vi "Finding Sensor Center.vi"() -> ()   [LabVIEW 2021]
uses:
  Classes/Workspace/Workspace.ctl
  Classes/Workspace/Component/Component Tray.lvclass
  Classes/Controller/Controller.lvclass
  Classes/Workspace/Fixture.lvclass
panel:
  out "error out":errorcluster
  in  "error in (no error)":errorcluster
  out "Workspace":T1
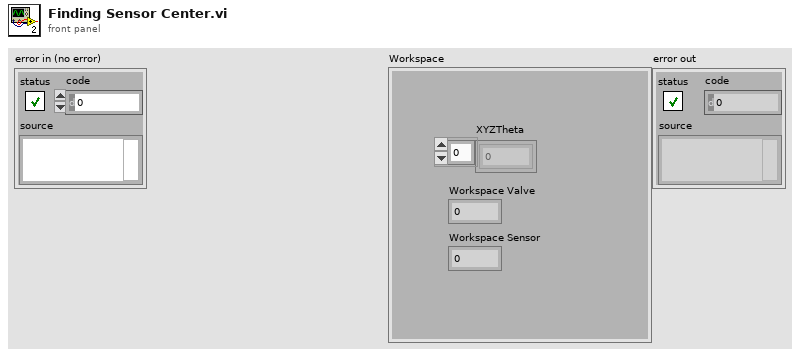
[diagram p1: front panel]
types:
  T1 = typedef "Fixture.lvclass/Workspace.ctl" = cluster{"XYZTheta":dbl[], "Workspace Valve":i32, "Workspace Sensor":i32}
  T2 = typedef "Controller.lvclass/Controllers.ctl" = cluster{"I-O.lvclass":refnum<class "I-O.lvclass">, "Gantry":refnum<k24>, "Dispenser":refnum<visa-resource-name>}
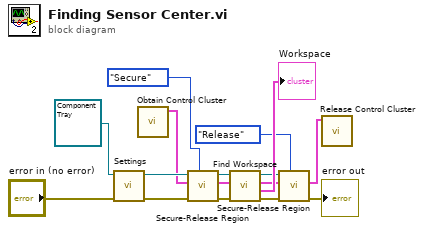
[diagram p0: block diagram]
diagram:
  n1 = call-dynamic "Settings.vi"("error in (no error)"="error in (no error)", "Component in"=refnum<class "Component Tray.lvclass"> refnum ("Component Tray.lvclass")) -> ("error out"=w4:errorcluster, "Component out"=w14:refnum<class "Component Tray.lvclass">)  [unwired: 8 in]
  n2 = call "Obtain Control Cluster.vi"() -> ("Control Out"=w11:T2)  [unwired: 11 in]
  n3 = call-dynamic "Secure-Release Region.vi"("Action"=enum16{"Secure", "Release"}."Secure", "error in (no error)"=w4, "Control In"=w11, "Workspace in"=w14) -> ("error out"=w3:errorcluster, "Control Out"=w10:T2, "Workspace out"=w9:refnum<class "Component Tray.lvclass">)  [unwired: 5 in]
  n4 = call-dynamic "Find Workspace.vi"("error in (no error)"=w3, "Control In"=w10, "Component.lvclass"=w9) -> ("error out"=w2:errorcluster, "Workspace"=→"Workspace":T1, "Control Out"=w7:T2, "Workspace Out"=w8:refnum<class "Component Tray.lvclass">)  [unwired: 5 in]
  n5 = call-dynamic "Secure-Release Region.vi"("Action"=enum16{"Secure", "Release"}."Release", "error in (no error)"=w2, "Control In"=w7, "Workspace in"=w8) -> ("error out"=→"error out":errorcluster, "Control Out"=w6:T2)  [unwired: 5 in, 1 out]
  n6 = call "Release Control Cluster.vi"("output cluster"=w6) -> ()  [unwired: 11 in]
